vi "Knock Signal Sim Test.vi"() -> ()   [LabVIEW 2013]
uses:
  IP Source/Knock Sensor/Generate Settings.ctl
  IP Source/APU/Input.ctl
  <vilib>/rvi/interface/RandomDataEmulation/nirviRandomDataOpen.vi
  <vilib>/rvi/interface/common/niFpgaCacheSessionInfoDynamic.vi
  <vilib>/rvi/interface/common/dynamic/niFpgaDynamicGetExecutionMode.vi
  <vilib>/FPGAPlugInAG/Dynamic/niLvFpga_Reset_Dynamic.vi
  <vilib>/rvi/interface/common/niFpgaWaitOnOcc.vi
  <vilib>/Utility/error.llb/Error Cluster From Error Code.vi
  <vilib>/rvi/errors/niLvFpgaAdjustHostInterfaceError.vi
  <vilib>/FPGAPlugInAG/Dynamic/niLvFpga_Run_Dynamic.vi
  <vilib>/FPGAPlugInAG/Dynamic/niLvFpga_Close_Dynamic.vi
  <vilib>/rvi/interface/nirviOpenFPGA/nirviOpenFPGA.xnode
  Simulation FPGA/APU + Knock.vi
  <vilib>/rvi/interface/nirviMethod/nirviMethod.xnode
  <vilib>/FPGA/interface/niFpgaViExecutionMode.ctl
  <vilib>/rvi/interface/nirviReadWriteControl/nirviReadWriteControl.xnode
  <vilib>/rvi/interface/nirviCloseFPGA/nirviCloseFPGA.xnode
  <vilib>/rvi/interface/Simulation/niFpgaSimulationCallBeginRW.vi
  IP Source/APU/APU.lvlib
  <vilib>/rvi/errors/niLvFpgaMergeErrorWithErrorCode.vi
  <vilib>/FPGAPlugInAG/Dynamic/niLvFpga_ReadFifo_Dynamic.vi
  NiFpgaLv.dll
  <vilib>/FPGAPlugInAG/Dynamic/niLvFpga_ConfigureFifo_Dynamic.vi
  <vilib>/FPGAPlugInAG/Dynamic/niLvFpga_StartFifo_Dynamic.vi
  <vilib>/FPGAPlugInAG/Dynamic/niLvFpga_StopFifo_Dynamic.vi
  IP Source/Knock Sensor/Knock Sensor.lvlib
panel:
  in  "input.Knock AO0":cluster{"low freq scaler":fxp<+,10,0>}={"low freq scaler"=0.099609375}
  out "Waveform Chart":cluster{dbl, i16}[](graph)=[{161.78466796875, 318}, {161.78466796875, 318}, {161.806640625, 318}, {161.806640625, 318}, {161.82861328125, 318}, {161.82861328125, 318}, {161.8505859375, 317}, {161.8505859375, 317}, {161.87255859375, 317}, {161.87255859375, 317}, {161.89453125, 317}, {161.89453125, 317}, {161.91650390625, 317}, {161.91650390625, 317}, {161.9384765625, 317}, {161.9384765625, 317}, {161.96044921875, 317}, {161.96044921875, 317}, {161.982421875, 316}, {161.982421875, 316}, {162.00439453125, 316}, {162.00439453125, 316}, {162.0263671875, 316}, {162.0263671875, 316}, {162.04833984375, 316}, {162.04833984375, 316}, {162.0703125, 315}, {162.0703125, 315}, {162.09228515625, 315}, {162.09228515625, 315}, {162.1142578125, 315}, {162.1142578125, 315}, {162.13623046875, 315}, {162.13623046875, 315}, {162.158203125, 314}, {162.158203125, 314}, {162.18017578125, 314}, {162.18017578125, 314}, {162.2021484375, 314}, {162.2021484375, 314}, {162.22412109375, 314}, {162.22412109375, 313}, {162.24609375, 313}, {162.24609375, 313}, {162.26806640625, 313}, {162.26806640625, 313}, {162.2900390625, 313}, {162.2900390625, 313}, {162.31201171875, 313}, {162.31201171875, 312}, {162.333984375, 312}, {162.333984375, 312}, {162.35595703125, 312}, {162.35595703125, 312}, {162.3779296875, 312}, {162.3779296875, 312}, {162.39990234375, 312}, {162.39990234375, 311}, {162.421875, 311}, {162.421875, 311}, {162.44384765625, 311}, {162.44384765625, 311}, {162.4658203125, 311}, {162.4658203125, 311}, {162.48779296875, 311}, {162.48779296875, 310}, {162.509765625, 310}]
  out "Timed Out?":bool
  in  "Cylinder Knock Configuration":T1(array[cluster])=[{"Trigger Angle"=0.0, "Probability"=100.0, "High Frequency Scaling Factor"=1.0}, {"Trigger Angle"=100.0, "Probability"=100.0, "High Frequency Scaling Factor"=0.75}, {"Trigger Angle"=250.0, "Probability"=100.0, "High Frequency Scaling Factor"=0.5}, {"Trigger Angle"=400.0, "Probability"=100.0, "High Frequency Scaling Factor"=0.25}]
  in  "Knock Configuration":T2={"low freq (periods/tick)"=0.0002500000409781933, "high freq (periods/tick)"=0.10000000009313226, "duration (1.25MHz tics)"=50.0, "low freq speed slope"=7.43865966796875e-05, "low freq speed intercept"=0.0, "low freq by speed"=FALSE} {"low freq speed slope" format="%.0g"}
  in  "RPM":dbl=5000000.0 format="%#_15g"
  in  "stop":bool
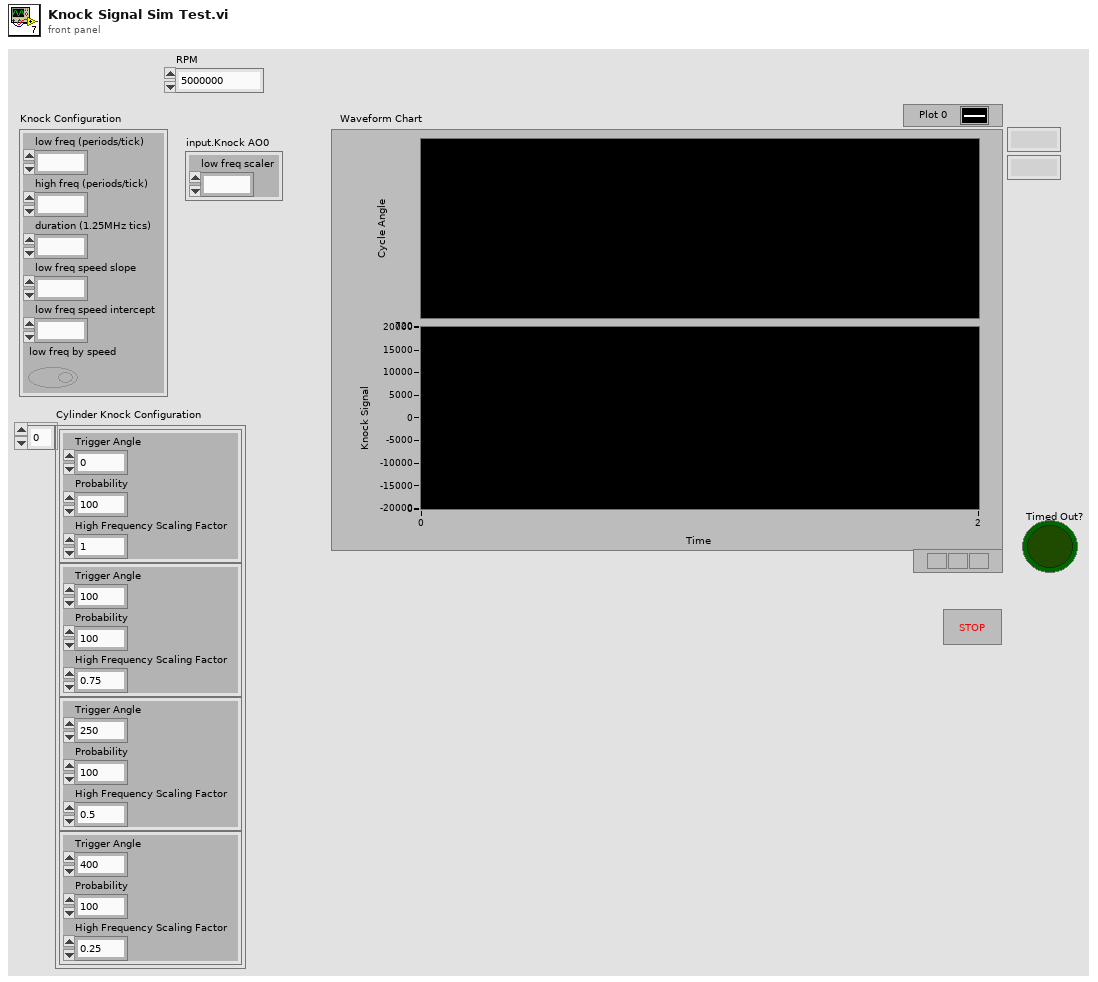
[diagram p1: front panel]
types:
  T1 = cluster{"Trigger Angle":dbl, "Probability":dbl, "High Frequency Scaling Factor":dbl}[]
  T2 = typedef "Engine Simulation Toolkit.lvlib/Knock Sensor.lvlib/Generate Settings.ctl" = cluster{"low freq (periods/tick)":fxp<+,32,0>, "high freq (periods/tick)":fxp<+,32,0>, "duration (1.25MHz tics)":fxp<+,18,18>, "low freq speed slope":fxp<+,16,-3>, "low freq speed intercept":fxp<+,10,-10>, "low freq by speed":bool}
  T3 = typedef "niFpgaViExecutionMode.ctl" = enum16{"FPGA Target", "Development Computer with Simulated I/O", "Development Computer with Real I/O", "Third-Party Simulator"}
  T4 = typedef "Engine Simulation Toolkit.lvlib/Knock Sensor.lvlib/Cylinder Input.ctl" = cluster{"probability compare":u16, "high freq scaler":fxp<+,10,0>, "trigger position":u16}
  T5 = typedef "Engine Simulation Toolkit.lvlib/Knock Sensor.lvlib/Cylinder Settings.ctl" = cluster{"seed":u16, "reset":bool}
  T6 = typedef "Engine Simulation Toolkit.lvlib/APU.lvlib/Input.ctl" = cluster{"desired speed":fxp<+/-,23,2>, "reset":bool}
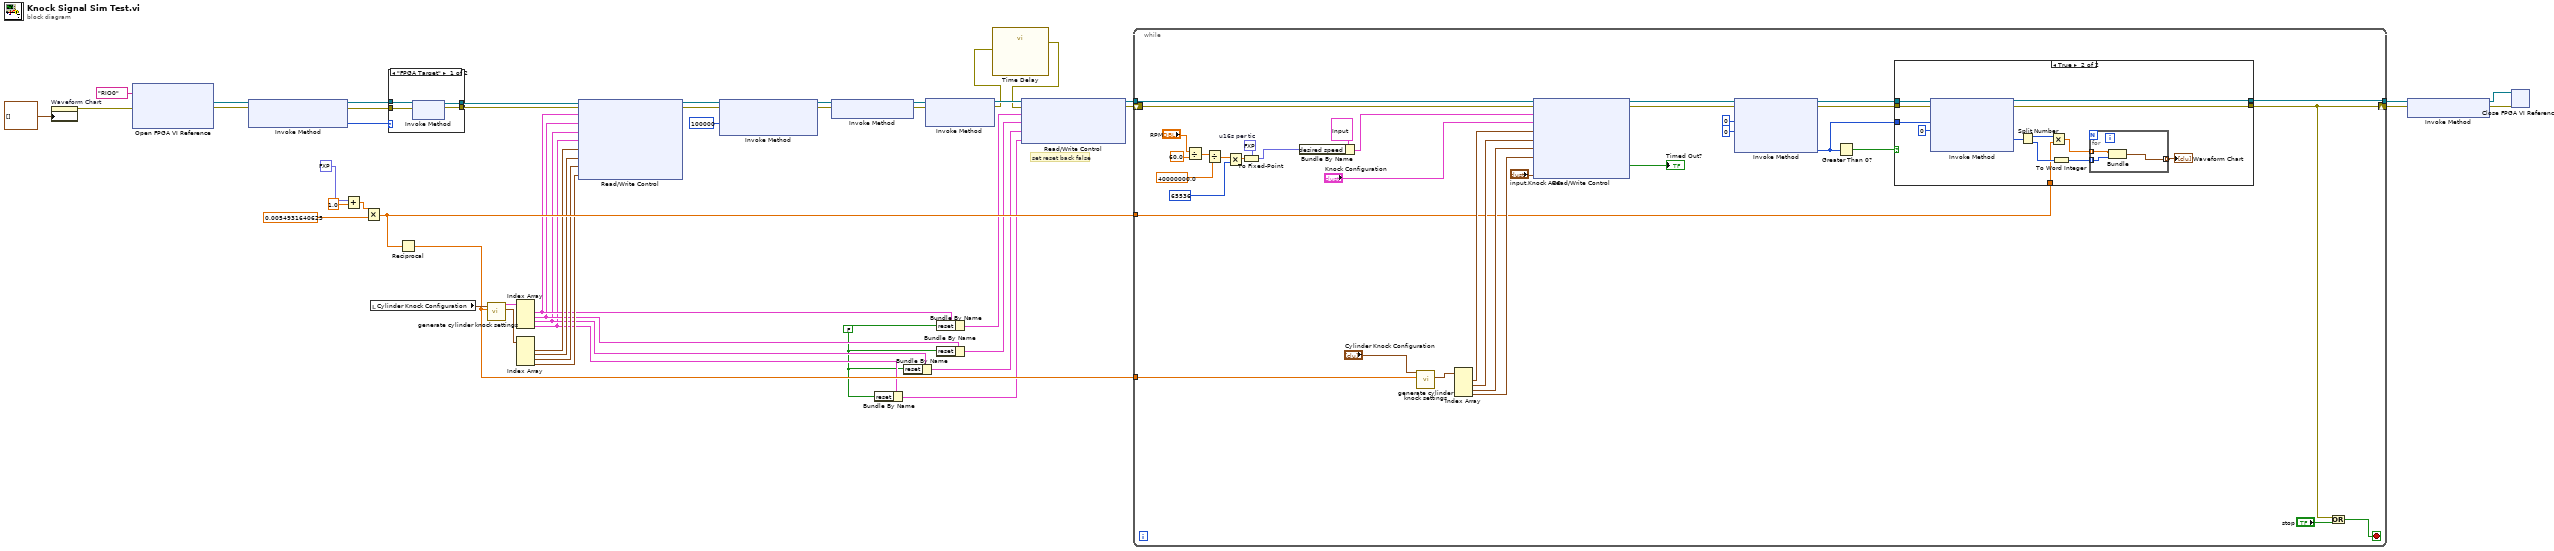
[diagram p0: block diagram]
diagram:
  w6 = FALSE
  # "set reset back false"
  n1 = property on="Waveform Chart" class="WFChart (strict)"("History Data"=cluster{dbl, i16}[] []) -> (error out=w23:errorcluster)  [unwired: 2 in, 1 out]
  n2 = xnode "Open FPGA VI Reference"("error in"=w23, "resource name"=tag "RIO0") -> ("FPGA VI Reference Out"=w47:refnum<k20>, "error out"=w31:errorcluster)
  n3 = xnode "Invoke Method"("FPGA VI Reference In"=w47, "error in"=w31) -> ("FPGA VI Reference Out"=w29:refnum<k20>, "error out"=w28:errorcluster, "FPGA VI Execution Mode"=w30:T3)
  n4 = Add(x=fxp<+,2,2> 1.0 ("extra cranks for a cycle"), y=1.0) -> (x+y=w46:dbl)
  n5 = Multiply(x=w46, y=0.0054931640625 ("x")) -> (x*y=w25:dbl)
  n6 = local read "Cylinder Knock Configuration"() -> (w42:T1)
  n7 = case shown="\"FPGA Target\"" w30 {
    tunnel: w29 -> [w52 w54]
    tunnel: w28 -> [w51 w53]
    tunnel: [w50 w54] -> w27
    tunnel: [w49 w53] -> w26
    frame "FPGA Target" {
      n8 = xnode "Invoke Method"("FPGA VI Reference In"=w52, "error in"=w51) -> ("FPGA VI Reference Out"=w50:refnum<k20>, "error out"=w49:errorcluster)
    }
    frame Default {
    }
  }
  n9 = Reciprocal(x=w25) -> (1/x=w24:dbl)
  n10 = call "generate cylinder knock settings.vi"("Convert Val"=w24, "Cylinder Knock Configuration"=w42) -> ("cylinder knock inputs"=w19:T4[], "Cylinder Knock Settings"=w41:T5[])  [unwired: 8 in]
  n11 = Index Array(array=w41) -> (element #1=w11:T5, element #2=w9:T5, element #3=w8:T5, element #4=w7:T5)  [unwired: 4 in]
  n12 = Index Array(array=w19) -> (element #1=w18:T4, element #2=w17:T4, element #3=w16:T4, element #4=w15:T4)  [unwired: 4 in]
  n13 = xnode "Read/Write Control"("FPGA VI Reference In"=w27, "error in"=w26, "settings.Knock AO0.Cylinder 1"=w11, "settings.Knock AO0.Cylinder 2"=w9, "settings.Knock AO0.Cylinder 3"=w8, "settings.Knock AO0.Cylinder 4"=w7, "input.Knock AO0.Cylinder 1"=w18, "input.Knock AO0.Cylinder 2"=w17, "input.Knock AO0.Cylinder 3"=w16, "input.Knock AO0.Cylinder 4"=w15) -> ("FPGA VI Reference Out"=w40:refnum<k20>, "error out"=w38:errorcluster)
  n14 = xnode "Invoke Method"("FPGA VI Reference In"=w40, "error in"=w38, "Requested Depth"=u32 100000) -> ("FPGA VI Reference Out"=w34:refnum<k20>, "error out"=w35:errorcluster)  [unwired: 1 out]
  n15 = xnode "Invoke Method"("FPGA VI Reference In"=w34, "error in"=w35) -> ("FPGA VI Reference Out"=w37:refnum<k20>, "error out"=w36:errorcluster)
  n16 = Bundle By Name(cluster=w7, "reset"=w6) -> (w3:T5)
  n17 = Bundle By Name(cluster=w8, "reset"=w6) -> (w4:T5)
  n18 = xnode "Invoke Method"("FPGA VI Reference In"=w37, "error in"=w36) -> ("FPGA VI Reference Out"=w12:refnum<k20>, "error out"=w2:errorcluster)  [unwired: 1 in]
  n19 = Bundle By Name(cluster=w11, "reset"=w6) -> (w10:T5)
  n20 = Bundle By Name(cluster=w9, "reset"=w6) -> (w5:T5)
  n21 = call "Time Delay"("error in (no error)"=w2) -> ("error out"=w1:errorcluster)  [unwired: 10 in]
  n22 = xnode "Read/Write Control"("FPGA VI Reference In"=w12, "error in"=w1, "settings.Knock AO0.Cylinder 1"=w10, "settings.Knock AO0.Cylinder 2"=w5, "settings.Knock AO0.Cylinder 3"=w4, "settings.Knock AO0.Cylinder 4"=w3) -> ("FPGA VI Reference Out"=w14:refnum<k20>, "error out"=w13:errorcluster)
  n23 = while {
    tunnel: w14 -> [w87]
    shift-right: [w60] -> w21
    shift-left: w13 -> [w88]
    tunnel: w25 -> [w57]
    tunnel: [w59] -> w20
    tunnel: w24 -> [w58]
    stop <- w89 stop-if-true
    w80 = fxp<+/-,23,2> 0.0  # u16s per tic
    n24 = Divide(x="RPM", y=60.0) -> (x/y=w85:dbl)
    n25 = Divide(x=w85, y=40000000.0) -> (x/y=w81:dbl)
    n26 = Multiply(x=w81, y=u32 65536 ("n")) -> (x*y=w79:dbl)
    n27 = To Fixed-Point(fixed-point type=w80, number=w79) -> (fixed-point=w78:fxp<+/-,23,2>)
    n28 = Bundle By Name(cluster=T6 {"desired speed"=0.0, "reset"=FALSE} ("my apu"), "desired speed"=w78) -> (w76:T6)
    n29 = call "generate cylinder knock settings.vi"("Convert Val"=w58, "Cylinder Knock Configuration"="Cylinder Knock Configuration") -> ("cylinder knock inputs"=w56:T4[])  [unwired: 8 in, 1 out]
    n30 = Index Array(array=w56) -> (element #1=w74:T4, element #2=w73:T4, element #3=w72:T4, element #4=w71:T4)  [unwired: 4 in]
    n31 = xnode "Read/Write Control"("FPGA VI Reference In"=w87, "error in"=w88, "Input.my apu"=w76, "settings.Knock AO0"="Knock Configuration", "input.Knock AO0.Cylinder 1"=w74, "input.Knock AO0.Cylinder 2"=w73, "input.Knock AO0.Cylinder 3"=w72, "input.Knock AO0.Cylinder 4"=w71, "input.Knock AO0"="input.Knock AO0") -> ("FPGA VI Reference Out"=w65:refnum<k20>, "error out"=w69:errorcluster, "Timed Out?"=→"Timed Out?":bool)
    n32 = xnode "Invoke Method"("FPGA VI Reference In"=w65, "error in"=w69, "Number of Elements"=u32 0, "Timeout (ms)"=0) -> ("FPGA VI Reference Out"=w63:refnum<k20>, "error out"=w62:errorcluster, "Elements Remaining"=w61:u32)  [unwired: 1 out]
    n33 = Greater Than 0?(x=w61) -> (x > 0?=w64:bool)
    n34 = case shown="True" w64 {
      tunnel: w63 -> [w91 w105]
      tunnel: w62 -> [w92 w104]
      tunnel: w61 -> [_ w103]
      tunnel: [w92 w101] -> w60
      tunnel: [w91 w100] -> w59
      tunnel: w57 -> [_ w96]
      frame False {
      }
      frame True {
        n35 = xnode "Invoke Method"("FPGA VI Reference In"=w105, "error in"=w104, "Number of Elements"=w103, "Timeout (ms)"=0) -> ("FPGA VI Reference Out"=w100:refnum<k20>, "error out"=w101:errorcluster, "Data"=w99:u32[])  [unwired: 1 out]
        n36 = Split Number(x=w99) -> (hi(x)=w94:u16[], lo(x)=w98:u16[])
        n37 = Multiply(x=w94, y=w96) -> (x*y=w95:dbl[])
        n38 = To Word Integer(number=w98) -> (16bit integer=w97:i16[])
        n39 = for {
          tunnel: w97 -> [w108] mode=indexing
          tunnel: [w107] -> w93 mode=indexing
          tunnel: w95 -> [w106] mode=indexing
          n40 = Bundle(w106, w108) -> (w107:cluster{dbl, i16})  [unwired: 1 in]
        }
        "Waveform Chart" <- w93
      }
    }
    n41 = Or(x=w60, y="stop") -> (x .or. y?=w89:bool)
  }
  n42 = xnode "Invoke Method"("FPGA VI Reference In"=w20, "error in"=w21) -> ("FPGA VI Reference Out"=w32:refnum<k20>, "error out"=w33:errorcluster)
  n43 = xnode "Close FPGA VI Reference"("FPGA VI Reference In"=w32, "error in"=w33) -> ()  [unwired: 1 out]
